vi "Centrifuge Tags.vi"(11 "AM Module Configs":T2[](array[typedef])) -> (1 "CM Tags":T1, 2 "CM Module Tags Array":T1[](array[typedef]), 3 "All Boolean Tags":string[](array[string]), 4 "All  Numeric Tags":string[](array[string]))   [LabVIEW 2018]
uses:
  Centrifuge Module Tag Names Cluster.ctl
  Centrifuge Module Config Cluster.ctl
  <vilib>/Utility/miscctls.llb/LVPoint32TypeDef.ctl
  Centrifuge Module Settings Cluster.ctl
  EPOS4/Controls/Device Selection.ctl
  EPOS4/Controls/EPOS Communication Settings.ctl
  Centrifuge Module.lvlib
  EPOS4/EPOS4.lvlib
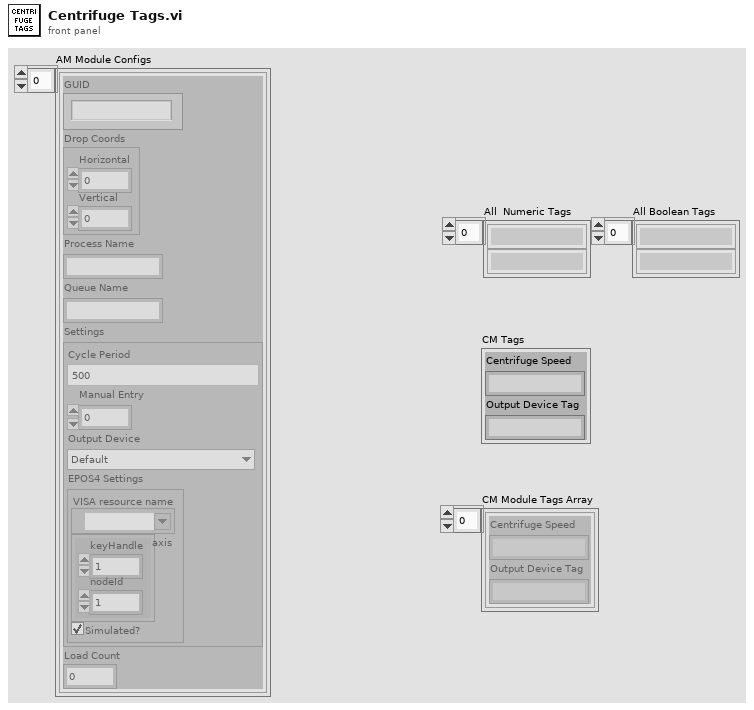
[diagram p1: front panel]
types:
  T1 = typedef "Centrifuge Module.lvlib/Centrifuge Module Tag Names Cluster.ctl" = cluster{"Centrifuge Speed":string, "Output Device Tag":string}
  T2 = typedef "Centrifuge Module.lvlib/Centrifuge Module Config Cluster.ctl" = cluster{"GUID":string, "Drop Coords":T3, "Process Name":string, "Queue Name":string, "Settings":T4, "Load Count":i32}
  T3 = typedef "LVPoint32TypeDef.ctl" = cluster{"Horizontal":i32, "Vertical":i32}
  T4 = typedef "Centrifuge Module.lvlib/Centrifuge Module Settings Cluster.ctl" = cluster{"Cycle Period":dbl, "Manual Entry":dbl, "Output Device":T5, "EPOS4 Settings":T6}
  T5 = typedef "Device Selection.ctl" = enum16{"Default", "EPOS4"}
  T6 = typedef "EPOS4.lvlib/EPOS Communication Settings.ctl" = cluster{"VISA resource name":refnum<visa-resource-name>, "axis":cluster{"keyHandle":u32, "nodeId":u16}, "Simulated?":bool}
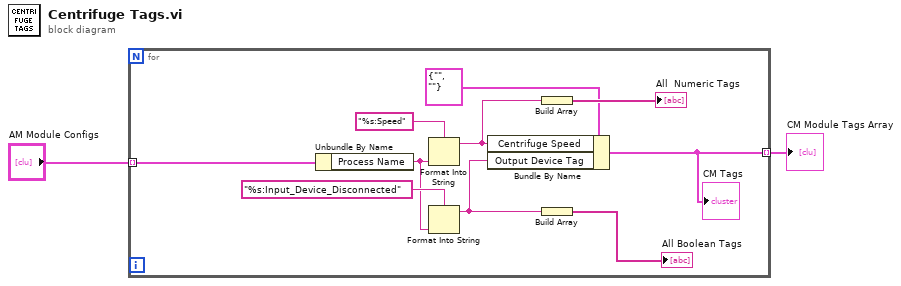
[diagram p0: block diagram]
diagram:
  n1 = for {
    tunnel: "AM Module Configs" -> [w6] mode=indexing
    tunnel: [w3] -> w1 mode=indexing
    n2 = Unbundle By Name(w6) -> ("Process Name"=w5:string)
    n3 = Format Into String(format string="%s:Speed", w5) -> (resulting string=w9:string)  [unwired: 2 in, 1 out]
    n4 = Format Into String(format string="%s:Input_Device_Disconnected", w5) -> (resulting string=w7:string)  [unwired: 2 in, 1 out]
    n5 = Bundle By Name(cluster=T1 {"Centrifuge Speed"="", "Output Device Tag"=""} ("Centrifuge Module Tag Names"), "Centrifuge Speed"=w9, "Output Device Tag"=w7) -> (w3:T1)
    "CM Tags" <- w3
    n6 = Build Array(w9) -> (→"All  Numeric Tags":string[])
    n7 = Build Array(w7) -> (→"All Boolean Tags":string[])
  }
  "CM Module Tags Array" <- w1
